vi "parse_MultiArrayLayout.vi"(4 "error in":errorcluster, 7 "msg in":string) -> (0 "error out":errorcluster, 1 "Data_Offset":u32, 2 "Array":T1, 3 "msg out":string)   [LabVIEW 2015]
uses:
  subs/parse_u32_scalar.vi
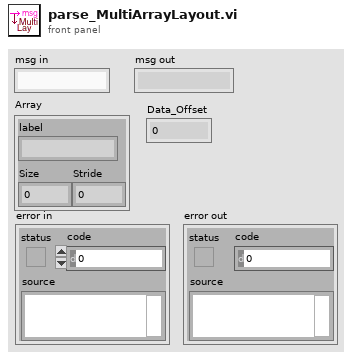
[diagram p1: front panel]
types:
  T1 = cluster{"label":string, "Size":u32, "Stride":u32}
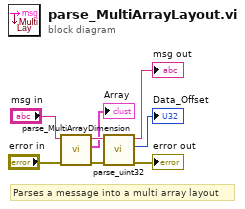
[diagram p0: block diagram]
diagram:
  # "Parses a message into a multi array layout"
  n1 = call "parse_MultiArrayDimension.vi"("error in"="error in", "msg in"="msg in") -> ("error out"=w5:errorcluster, "Array"=→"Array":T1, "msg out"=w6:string)  [unwired: 3 in]
  n2 = call-poly "parse_uint32.vi"("error in"=w5, "msg in"=w6) -> ("error out"=→"error out":errorcluster, "number"=→"Data_Offset":u32, "msg out"=→"msg out":string)  [unwired: 3 in]
